vi "releasebuff.vi"(6 "slock too?":bool, 8 "error in":errorcluster, 9 "pointer":u64, 10 "buffer name":string, 11 "Buffers":T1[](array[typedef])) -> (0 "error out":errorcluster, 1 "is locked":bool, 2 "output buffer":T1, 3 "Buffers out":T1[](array[typedef]))   [LabVIEW 2016]
uses:
  private/vis/BufferStruct.ctl
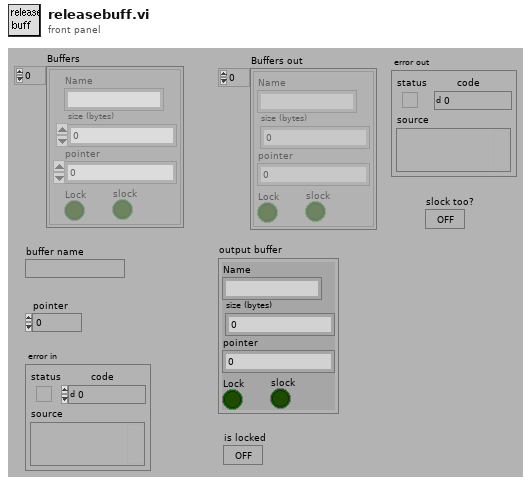
[diagram p1: front panel]
types:
  T1 = typedef "BufferStruct.ctl" = cluster{"Name":string, "size (bytes)":u64, "pointer":u64, "Lock":bool, "slock":bool}
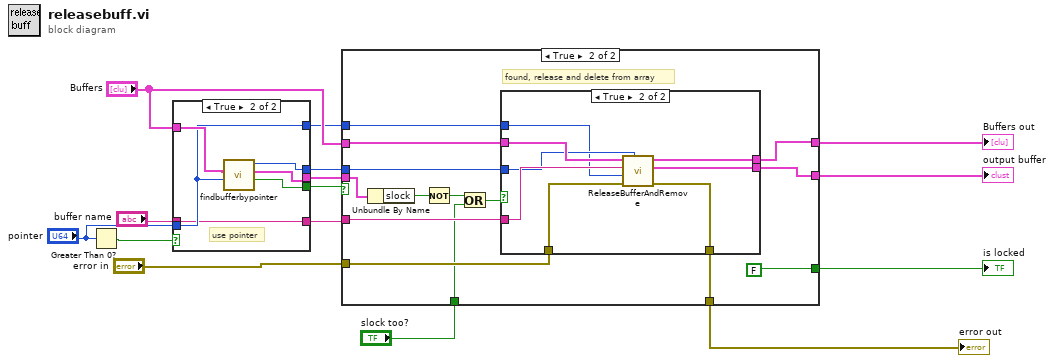
[diagram p0: block diagram]
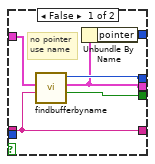
[diagram p2: hidden frame]
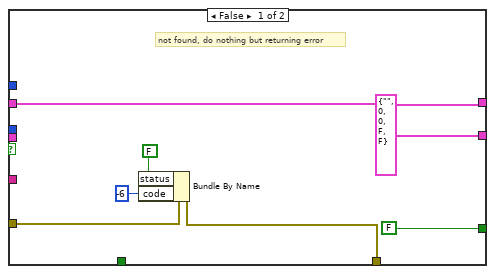
[diagram p3: hidden frame]
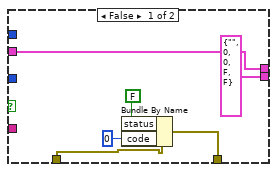
[diagram p4: hidden frame]
diagram:
  n1 = Greater Than 0?(x="pointer") -> (x > 0?=w6:bool)
  n2 = case shown="True" w6 {
    tunnel: [w21 w24] -> w10
    tunnel: "Buffers" -> [w20 w27]
    tunnel: [w17 w25] -> w9
    tunnel: [w19 w26] -> w8
    tunnel: "buffer name" -> [w18 w22]
    tunnel: [w18 w22] -> w4
    tunnel: [w16 w23] -> w3
    tunnel: "pointer" -> [_ w23]
    frame False {
      # "no pointer\nuse name"
      n3 = call "findbufferbyname.vi"("buffer name"=w18, "Buffers"=w20) -> ("found"=w19:bool, "buffer found"=w17:T1, "index"=w21:i32)  [unwired: 7 out]
      n4 = Unbundle By Name(w17) -> ("pointer"=w16:u64)
    }
    frame True {
      # "use pointer"
      n5 = call "findbufferbypointer.vi"("pointer"=w23, "Buffers"=w27) -> ("found"=w26:bool, "buffer found"=w25:T1, "index"=w24:i32)  [unwired: 7 out]
    }
  }
  n6 = case shown="True" w8 {
    tunnel: w9 -> [_ w39]
    tunnel: w4 -> [_ w46]
    tunnel: "Buffers" -> [w34 w47]
    tunnel: [w34 w42] -> w11
    tunnel: w10 -> [_ w41]
    tunnel: [T1 {"Name"="", "size (bytes)"=0, "pointer"=0, "Lock"=FALSE, "slock"=FALSE} ("output buffer") w43] -> w12
    tunnel: [FALSE ("is locked") FALSE ("is locked")] -> w13
    tunnel: "error in" -> [w32 w45]
    tunnel: [w31 w44] -> w15
    tunnel: w3 -> [_ w40]
    tunnel: "slock too?" -> [_ w38]
    frame False {
      # "not found, do nothing but returning error"
      n7 = Bundle By Name(cluster=w32, "status"=FALSE, "code"=-6) -> (w31:errorcluster)
    }
    frame True {
      # "found, release and delete from array"
      n8 = Unbundle By Name(w39) -> ("slock"=w36:bool)
      n9 = Not(x=w36) -> (.not. x?=w35:bool)
      n10 = Or(x=w35, y=w38) -> (x .or. y?=w37:bool)
      n11 = case shown="True" w37 {
        tunnel: w47 -> [w54 w62]
        tunnel: w46 -> [_ w61]
        tunnel: w45 -> [w50 w60]
        tunnel: [w49 w59] -> w44
        tunnel: [T1 {"Name"="", "size (bytes)"=0, "pointer"=0, "Lock"=FALSE, "slock"=FALSE} ("output buffer") w58] -> w43
        tunnel: [w54 w57] -> w42
        tunnel: w41 -> [_ w56]
        tunnel: w40 -> [_ w55]
        frame False {
          n12 = Bundle By Name(cluster=w50, "status"=FALSE, "code"=0) -> (w49:errorcluster)
        }
        frame True {
          n13 = call "ReleaseBufferAndRemove.vi"("index"=w56, "error in (no error)"=w60, "pointer"=w55, "Buffer Name"=w61, "Buffers"=w62) -> ("error out"=w59:errorcluster, "output buffer"=w58:T1, "output buffers"=w57:T1[])  [unwired: 4 out]
        }
      }
    }
  }
  "error out" <- w15
  "is locked" <- w13
  "output buffer" <- w12
  "Buffers out" <- w11
